vi "Chirp Z Transform (CDB).vi"(6 "algorithm":u16(ring)=1 items=["direct", "frequency domain"], 8 "increment":cdb=1.0+0.0i, 9 "starting point":cdb=1.0+0.0i, 10 "# of bins":i32=-1, 11 "X":cdb[](array[numeric])) -> (0 "error":i32, 3 "Chirp-Z {X}":cdb[](array[numeric]))   [LabVIEW 2018, in "NI_AALPro.lvlib"]
doc: "Computes the Chirp-Z transform of the input sequence <B>X</B>. Wire data to the <B>X</B> input to determine the polymorphic instance to use or manually select the instance."
uses:
  NI_AALPro.lvlib
  <resource>/lvanlys.dll
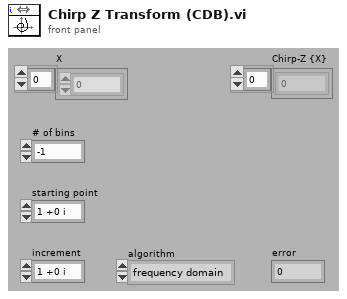
[diagram p1: front panel]
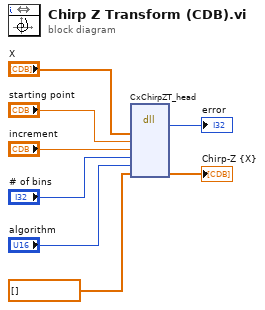
[diagram p0: block diagram]
diagram:
  n1 = dll-call lib="C:/Program Files (x86)/National Instruments/LabVIEW 2018/resource/lvanlys.*" fn="CxChirpZT_head"("X"="X", "starting point"="starting point", "increment"="increment", "samples"="# of bins", "algorithm"="algorithm", "Chirp Z {X}"=cdb[] []) -> (→"error":i32, "Chirp Z {X}"=→"Chirp-Z {X}":cdb[])  [unwired: 8 in, 2 out]
